vi "Calculate Round Score.vi"(1 "My Move":T1, 2 "Opponent's Move":T1) -> (0 "Round Score":u32)   [LabVIEW 2020, in "AoC 2022.lvlib"]
uses:
  AoC 2022.lvlib
  Play Item.ctl
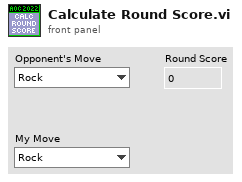
[diagram p1: front panel]
types:
  T1 = typedef "AoC 2022.lvlib/Play Item.ctl" = enum16{"Rock", "Paper", "Scissor"}
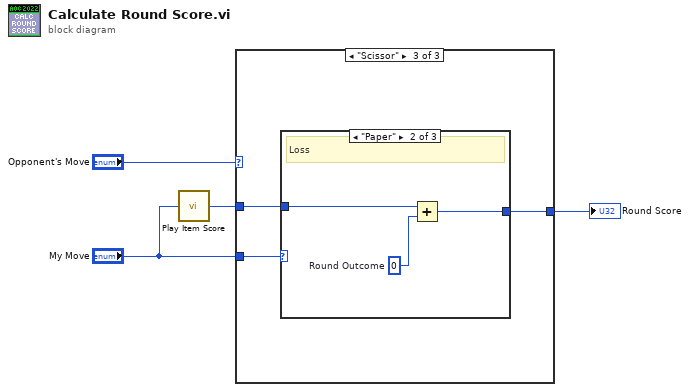
[diagram p0: block diagram]
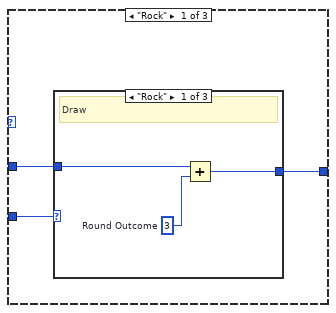
[diagram p2: hidden frame]
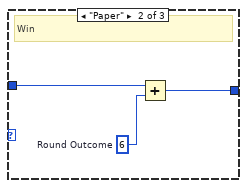
[diagram p3: hidden frame]
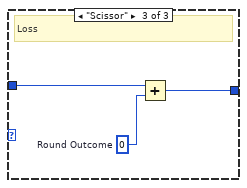
[diagram p4: hidden frame]
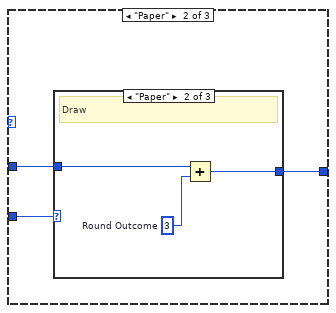
[diagram p5: hidden frame]
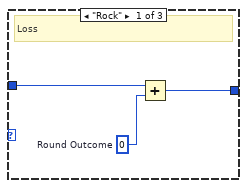
[diagram p6: hidden frame]
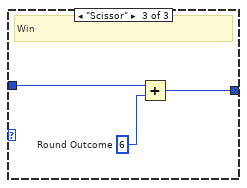
[diagram p7: hidden frame]
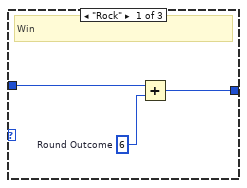
[diagram p8: hidden frame]
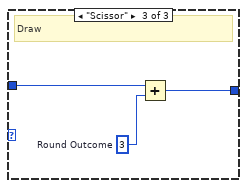
[diagram p9: hidden frame]
diagram:
  n1 = call "Play Item Score.vi"("Play Item"="My Move") -> ("Score"=w3:u32)  [unwired: 4 in]
  n2 = case shown="\"Scissor\"" "Opponent's Move" {
    tunnel: "My Move" -> [w7 w19 w31]
    tunnel: w3 -> [w6 w18 w30]
    tunnel: [w5 w17 w29] -> w4
    frame "Rock" {
      n3 = case shown="\"Rock\"" w7 {
        tunnel: w6 -> [w8 w11 w14]
        tunnel: [w10 w13 w16] -> w5
        frame "Rock" {
          w9 = u32 3  # Round Outcome
          # "Draw"
          n4 = Add(x=w8, y=w9) -> (x+y=w10:u32)
        }
        frame "Paper" {
          w12 = u32 6  # Round Outcome
          # "Win"
          n5 = Add(x=w11, y=w12) -> (x+y=w13:u32)
        }
        frame "Scissor" {
          w15 = u32 0  # Round Outcome
          # "Loss"
          n6 = Add(x=w14, y=w15) -> (x+y=w16:u32)
        }
      }
    }
    frame "Paper" {
      n7 = case shown="\"Paper\"" w19 {
        tunnel: w18 -> [w20 w23 w26]
        tunnel: [w22 w25 w28] -> w17
        frame "Rock" {
          w21 = u32 0  # Round Outcome
          # "Loss"
          n8 = Add(x=w20, y=w21) -> (x+y=w22:u32)
        }
        frame "Paper" {
          w24 = u32 3  # Round Outcome
          # "Draw"
          n9 = Add(x=w23, y=w24) -> (x+y=w25:u32)
        }
        frame "Scissor" {
          w27 = u32 6  # Round Outcome
          # "Win"
          n10 = Add(x=w26, y=w27) -> (x+y=w28:u32)
        }
      }
    }
    frame "Scissor" {
      n11 = case shown="\"Paper\"" w31 {
        tunnel: w30 -> [w32 w35 w38]
        tunnel: [w34 w37 w40] -> w29
        frame "Rock" {
          w33 = u32 6  # Round Outcome
          # "Win"
          n12 = Add(x=w32, y=w33) -> (x+y=w34:u32)
        }
        frame "Paper" {
          w36 = u32 0  # Round Outcome
          # "Loss"
          n13 = Add(x=w35, y=w36) -> (x+y=w37:u32)
        }
        frame "Scissor" {
          w39 = u32 3  # Round Outcome
          # "Draw"
          n14 = Add(x=w38, y=w39) -> (x+y=w40:u32)
        }
      }
    }
  }
  "Round Score" <- w4
